vi "Cache-GlobalEventQueues.vi"(6 "Create? (F)":bool, 8 "error in (no error)":errorcluster) -> (0 "error out":errorcluster, 2 "CreatedQueue":refnum<queue>, 3 "Queue":refnum<queue>[](array[refnum]))   [LabVIEW 2017, in "Communicable State Machine.lvlib"]
doc: "-- <b>Controls</b> --\n- <b>Create(F)</b>:\n\n-- <b>Indicators</b> --\n- <b>CSM Global Log Event</b>:"
uses:
  Communicable State Machine.lvlib
  Typedef/_CSM_GlobalLog_MSG.ctl
  Typedef/_CSM_Response Source Message.ctl
  Typedef/_CSM_GlobalLog_MSG_TYPE.ctl
  ChangeFlag/ChangeFlag-Write.vi
  Utility/Random Change Flag.vi
  ChangeFlag/ChangeFlagDB.vi
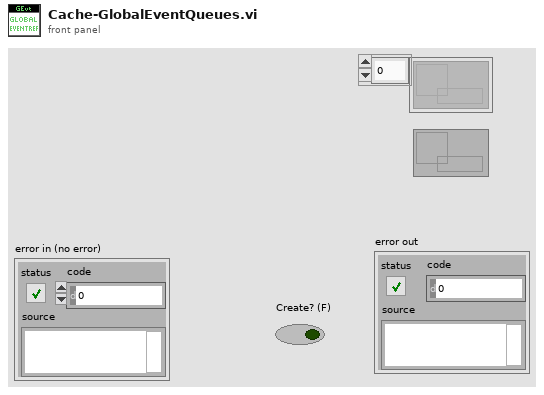
[diagram p1: front panel]
types:
  T1 = typedef "Communicable State Machine.lvlib/_CSM_GlobalLog_MSG.ctl" = cluster{"Name (\"\" to Use UUID)":string, "Current State":string, "Arguments":string, "Source Message":T2, "Source Module":string, "Complete(T)/Start(F)":bool, "LogType":T3, "Time Stamp":timestamp}
  T2 = typedef "Communicable State Machine.lvlib/_CSM_Response Source Message.ctl" = cluster{"‘State":string, "’Arguments":string, "’Error":errorcluster}
  T3 = typedef "Communicable State Machine.lvlib/_CSM_GlobalLog_MSG_TYPE.ctl" = enum16{"User Log", "State Change", "Status", "Interrupt", "Register", "Unregister", "Error Log", "Module Created", "Module Destroyed"}
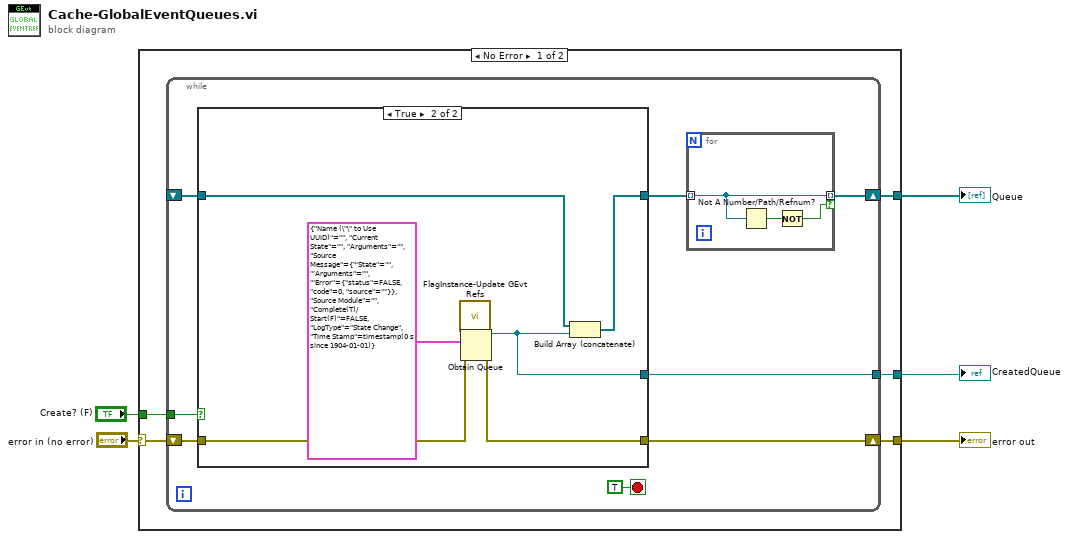
[diagram p0: block diagram]
diagram:
  n1 = case shown="No Error" "error in (no error)" {
    selector: "error in (no error)" -> [w9 w30]
    tunnel: [w10 _] -> w5
    tunnel: [w8 w30] -> w3
    tunnel: "Create? (F)" -> [w7 _]
    tunnel: [w6 _] -> w1
    frame No Error {
      n2 = while {
        shift-right: [w17] -> w8
        shift-left: w9 -> [w18]
        shift-right: [w12] -> w10
        shift-left: _ -> [w15]
        tunnel: w7 -> [w14]
        tunnel: [w13] -> w6
        stop <- TRUE stop-if-true
        n3 = case shown="True" w14 {
          tunnel: [w23 w27] -> w11
          tunnel: w18 -> [w22 w28]
          tunnel: [w22 w29] -> w17
          tunnel: w15 -> [w23 w24]
          tunnel: [_ w25] -> w13
          frame False {
          }
          frame True {
            n4 = call "FlagInstance-Update GEvt Refs.vi"() -> ()  [unwired: 10 in, 2 out]
            n5 = Obtain Queue(element data type=T1 {"Name (\"\" to Use UUID)"="", "Current State"="", "Arguments"="", "Source Message"={"‘State"="", "’Arguments"="", "’Error"={"status"=FALSE, "code"=0, "source"=""}}, "Source Module"="", "Complete(T)/Start(F)"=FALSE, "LogType"=enum."State Change", "Time Stamp"=timestamp(0 s since 1904-01-01)} ("Cross JKI State Machine Data"), error in (no error)=w28) -> (queue out=w25:refnum<queue>, error out=w29:errorcluster)  [unwired: 3 in, 1 out]
            n6 = Build Array (concatenate)(w24, w25) -> (w27:refnum<queue>[])
          }
        }
        n7 = for {
          tunnel: [w21] -> w12 mode=indexing if=w19
          tunnel: w11 -> [w21] mode=indexing
          n8 = Not A Number/Path/Refnum?(number/path/refnum=w21) -> (NaN/Path/Refnum?=w20:bool)
          n9 = Not(x=w20) -> (.not. x?=w19:bool)
        }
      }
    }
    frame Error {
    }
  }
  "Queue" <- w5
  "error out" <- w3
  "CreatedQueue" <- w1
